vi "Main.vi"() -> ()   [LabVIEW 2018]
panel:
  out "Array":dbl[](array[numeric])
  out "Cont em Seg":dbl caption="Contador em Segundos"
  out "Regressive Timer":i32
  out "Case Indicator":i8
  out "Cont Min":dbl caption="Contador em Minutos"
  in  "stop":bool
  out "Barramento":string
  in  "Tab Control":T1(tab)
  in  "Rampa 1":i8=50 min=0 max=80 step=1
  in  "Fechamento \nde Enzimas":i8 min=0 max=80 step=1
  in  "Iniciar":bool
  in  "Min L3":i32 min=0 step=1
  in  "Min L2":i32 min=0 step=1
  in  "Min L1":i32 min=0 step=1
  in  "Min Ferv":i32 min=0 step=1
  in  "Qt de \nLupulos":i8 min=0 max=3 step=1
  in  "Min FE":i32 min=0 step=1
  in  "Min R4":i32 min=0 step=1
  in  "Min R3":i32 min=0 step=1
  in  "Min R2":i32 min=0 step=1
  in  "Min R1":i32 min=0 step=1
  in  "Qt de Rampas":i8 min=0 max=4 step=1
  in  "Rampa 4":i8 min=0 max=80 step=1
  in  "Rampa 3":i8 min=0 max=80 step=1
  in  "Rampa 2":i8 min=0 max=80 step=1
  out "Waveform Graph":dbl[](graph)
  in  "Set B1":bool
  in  "Chv Manual Most":bool
  in  "Slide Pot Most":i8(slide)=19 min=0 max=100 scale=0.0..100.0
  out "Led Manual Most":bool
  out "Seg Prox R":i8
  out "Min Prox R":i8
  out "Status Misturador Most":bool
  out "Porcent Pot Most":dbl
  out "Rampa Atual":string
  out "SetPoint Temp":dbl
  out "Seg Most":dbl
  out "Min Most":dbl
  out "Hora Most":dbl
  out "Watts Pot Most":dbl
  out "Thermometer Most":dbl(slide) caption="TMost" scale=0.0..100.0
  out "Status Resistencia Most":bool
  out "Lúpulo 1":bool
  out "Lúpulo 2":bool
  out "Lúpulo 3":bool
  out "Rampa 1":bool
  out "Rampa 2":bool
  out "Rampa 3":bool
  out "Rampa 4":bool
  out "Fech de Enzimas":bool
  out "Fervura":bool
  out "Transferência":bool
  out "Mosturação":bool
  out "Setup":bool
  in  "Iniciar 2":bool
  in  "Resistencia":bool
  in  "Misturador":bool
  in  "Bomba":bool
  in  "Set B2":bool
  out "Porcent Pot Ferv":dbl
  in  "Chv Manual Ferv":bool
  out "Led Manual Ferv":bool
  in  "Slide Pot Ferv":i8(slide) min=0 max=100 step=1 scale=0.0..100.0
  out "Thermometer Ferv":dbl(slide) scale=0.0..100.0
  out "Botão Lupulo 3":bool
  out "Botão Lupulo 2":bool
  out "Botão Lupulo 1":bool
  out "Status Resistencia Ferv":bool
  out "Watts Pot Ferv":dbl
  out "Min Prox L":i32
  out "Seg Prox L":i32
  out "Hora Ferv":dbl
  out "Min Ferv":dbl
  out "Seg Ferv":dbl
  # "Processo de cerveja artesanal automatizado"
  # "Rampas de Temperatura"
  # "Tempo nas respectivas rampas"
  # "Tempo de fervura"
  # "ºC"
  # "1ª Rampa :"
  # "Minutos"
  # "Minutos"
  # "ºC"
  # "Minutos"
  # "2ª Rampa :"
  # "Tempo dos lúpulos"
  # "Minutos"
  # "ºC"
  # "Minutos"
  # "3ª Rampa :"
  # "Minutos"
  # "ºC"
  # "Minutos"
  # "4ª Rampa :"
  # "Rampas Temperatura"
  # "Minutos"
  # "Fechamento Enzimas :"
  # "Quantidade de Lúpulos"
  # "ºC"
  # "Minutos"
  # "Controle Manual"
  # "Temperatura (ºC)"
  # "Controle Supervisório :"
  # "Misturador :"
  # "Resistência :"
  # "Potência da Resistência :"
  # "W"
  # "Porcentagem Potência :"
  # "%"
  # "Rampa atual :"
  # "Valor da Rampa Atual :"
  # "ºC"
  # "Tempo p/ próxima rampa :"
  # "m"
  # "s"
  # "Tempo de Processo :"
  # "h"
  # "m"
  # "s"
  # "Bomba de Recirculação"
  # "Misturador"
  # "Resistência"
  # "Etapas Fervura"
  # "Etapas Mosturação"
  # "Processo Atual"
  # "Controle Manual"
  # "Controle Supervisório :"
  # "Temperatura (ºC)"
  # "Resistência :"
  # "Potência da Resistência :"
  # "W"
  # "Porcentagem Potência :"
  # "%"
  # "Lúpulo 1"
  # "Lúpulo 2"
  # "Lúpulo 3"
  # "Tempo p/ próximo lúpulo :"
  # "m"
  # "s"
  # "Tempo de Processo :"
  # "s"
  # "m"
  # "h"
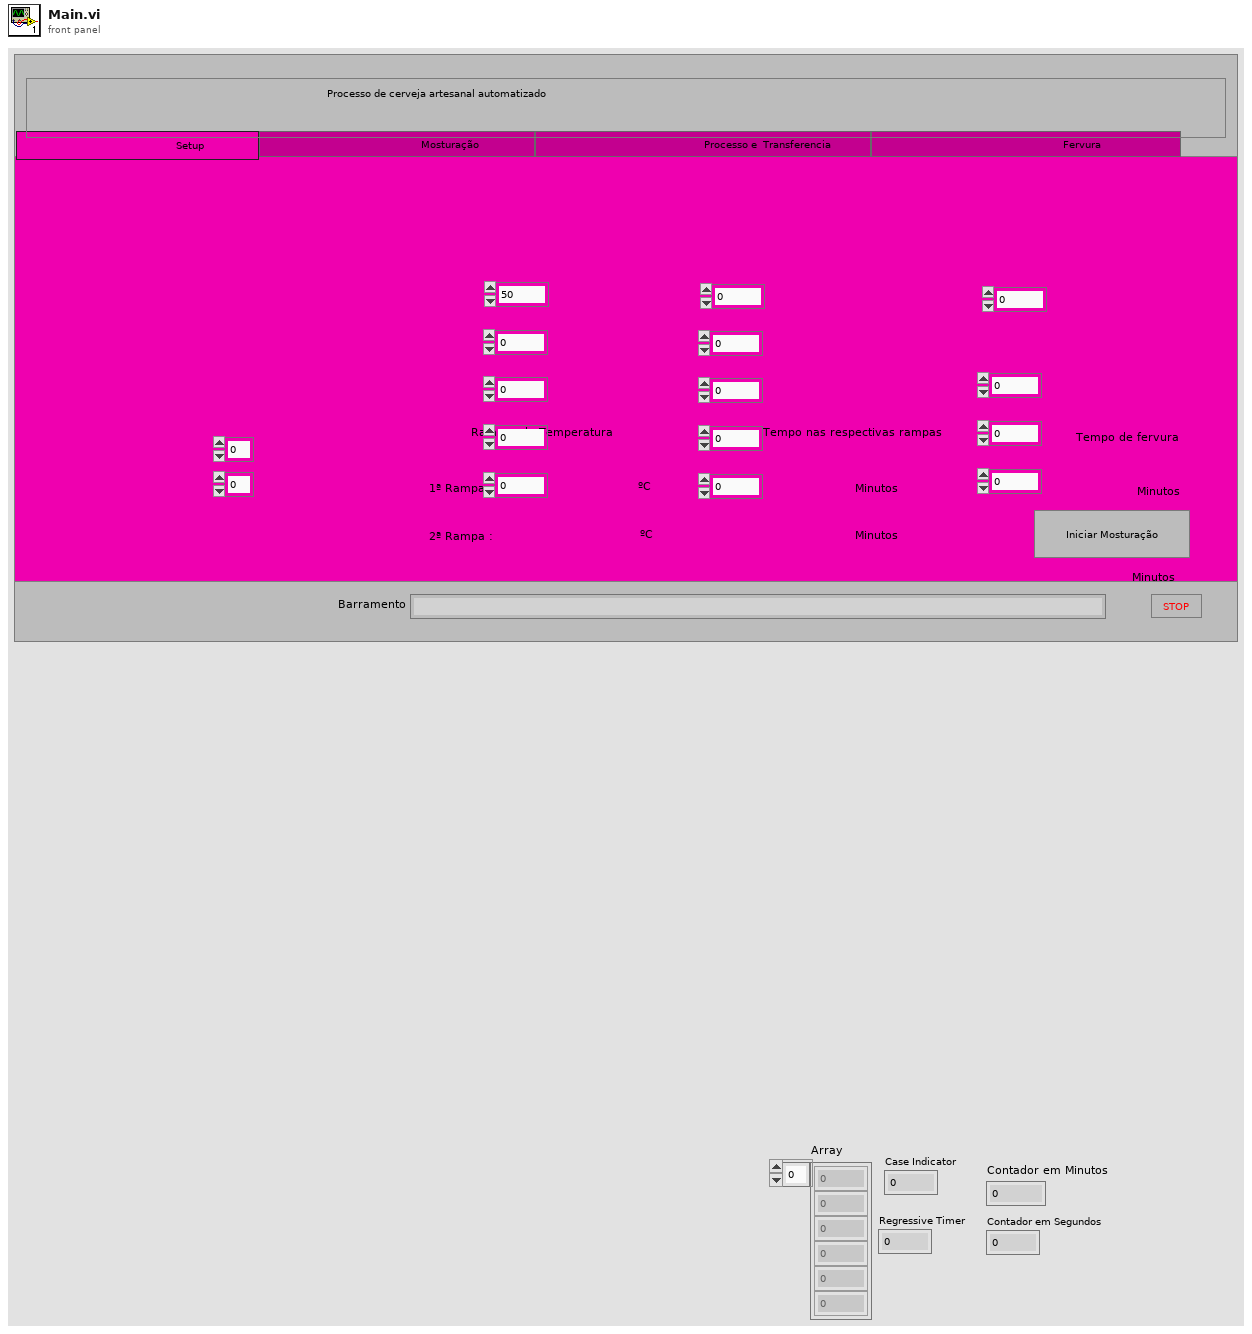
[diagram p1: front panel]
types:
  T1 = enum32{"                                   Setup                                ", "                                   Mosturação                                 ", "                                           Processo e  Transferencia                      ", "                                     Fervura                                                 "}
  T2 = typedef "LVDateTimeRec.ctl" = cluster{"fractional second":dbl, "second":i32, "minute":i32, "hour":i32, "day of month":i32, "month":i32, "year":i32, "day of week":i32, "day of year":i32, "DST":i32}
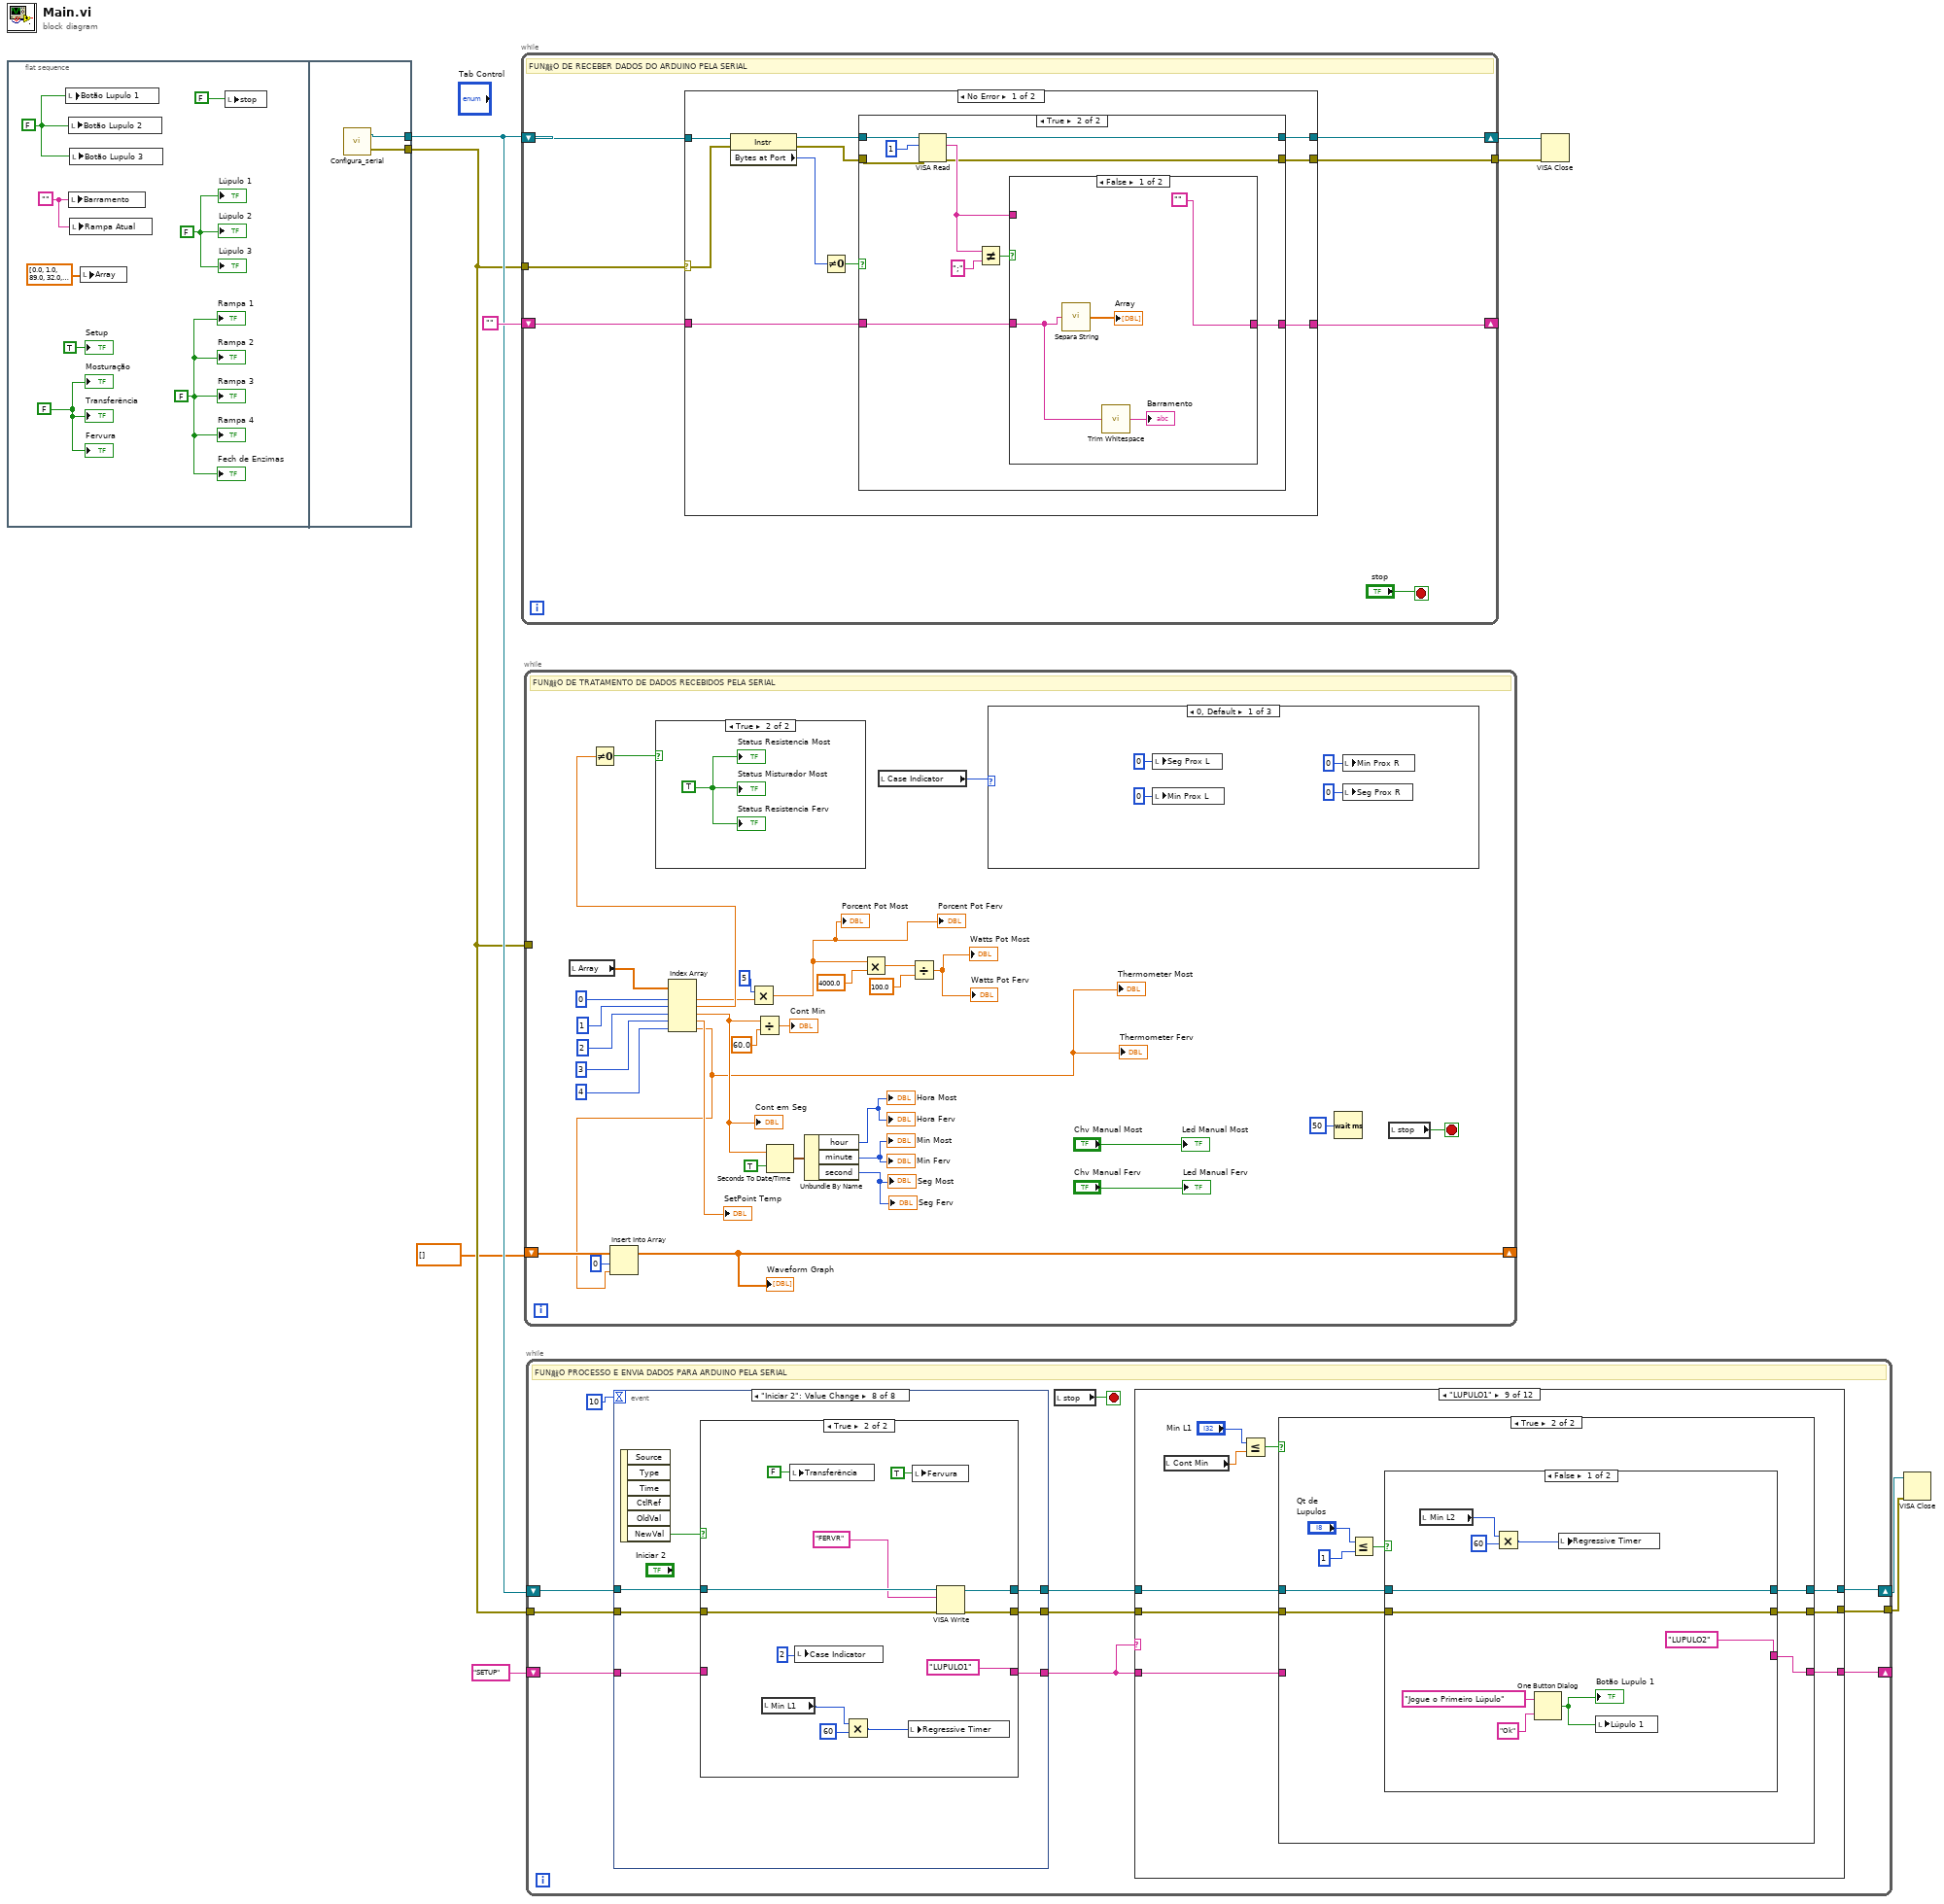
[diagram p0: block diagram]
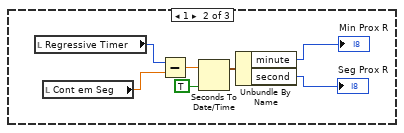
[diagram p2: hidden frame]
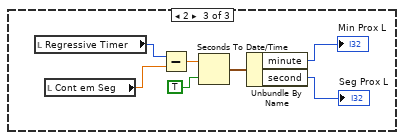
[diagram p3: hidden frame]
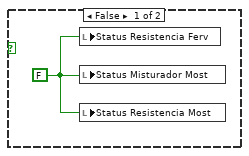
[diagram p4: hidden frame]
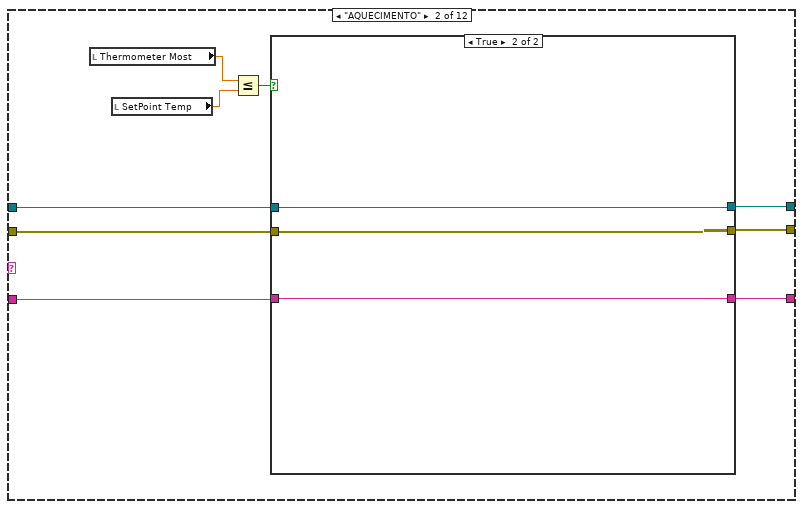
[diagram p6: hidden frame]
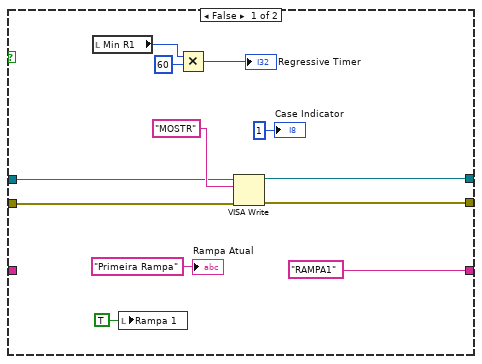
[diagram p7: hidden frame]
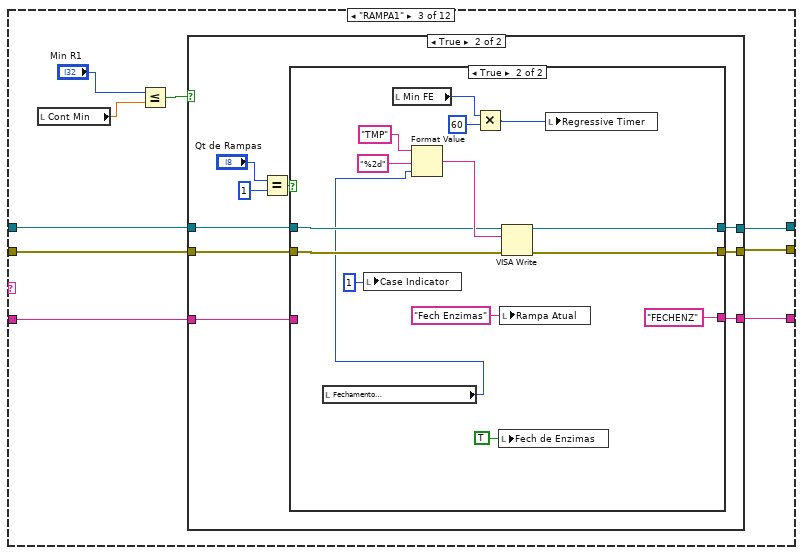
[diagram p8: hidden frame]
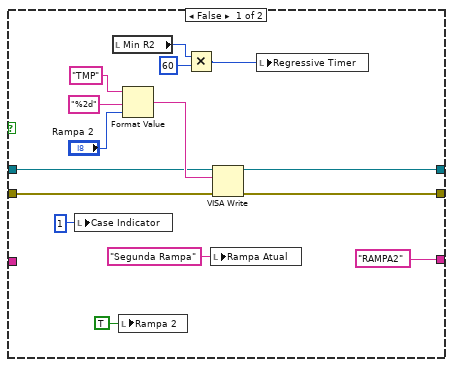
[diagram p10: hidden frame]
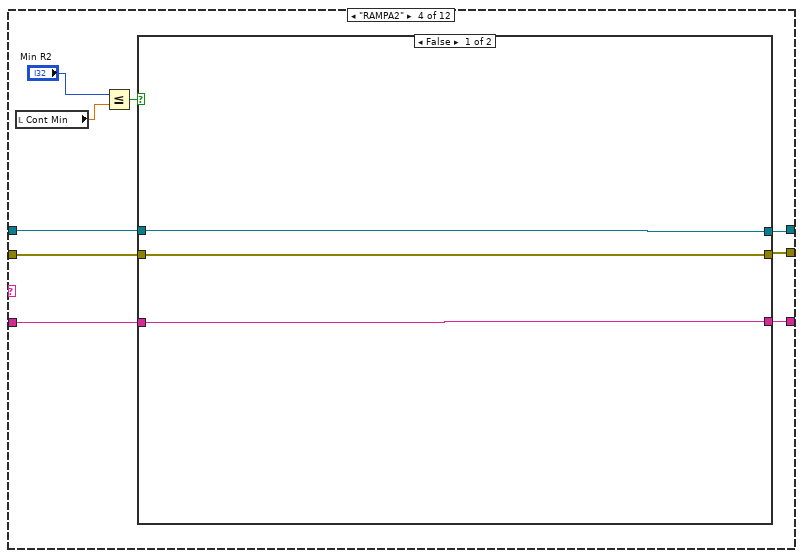
[diagram p11: hidden frame]
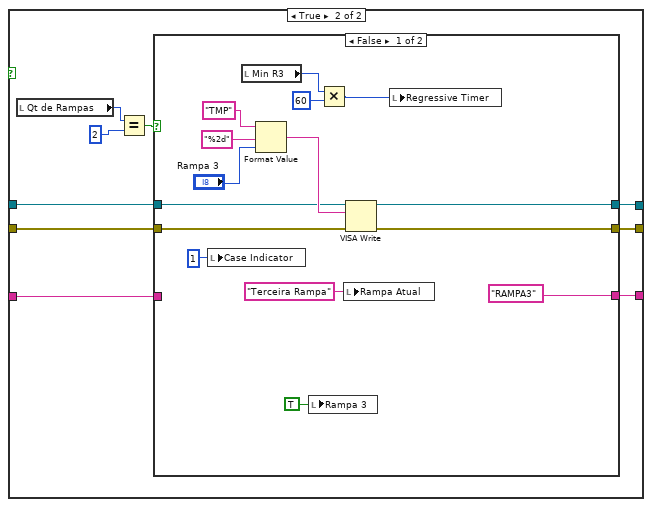
[diagram p12: hidden frame]
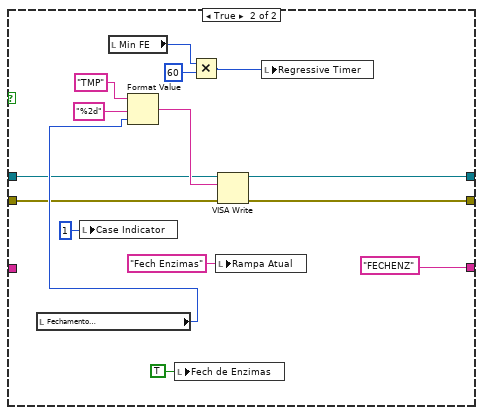
[diagram p13: hidden frame]
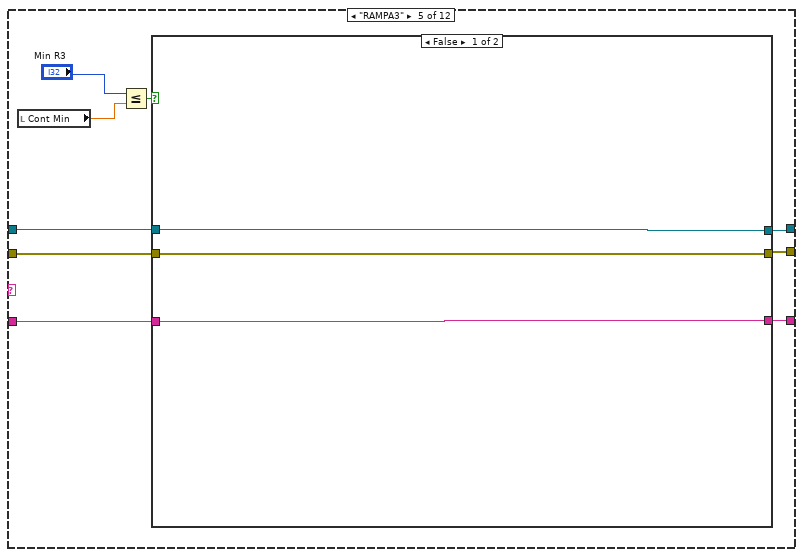
[diagram p14: hidden frame]
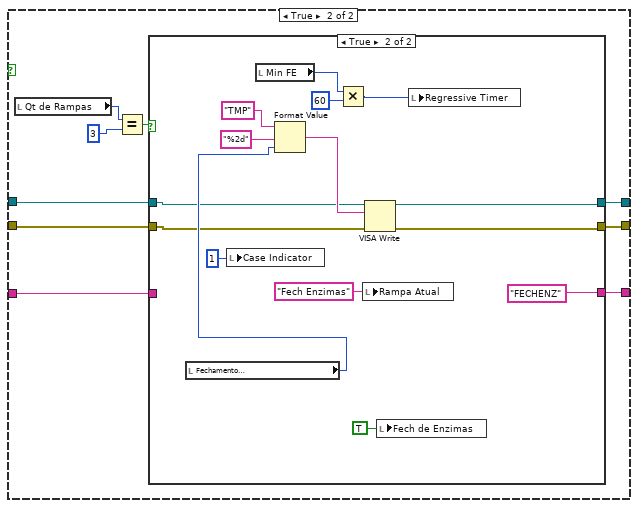
[diagram p15: hidden frame]
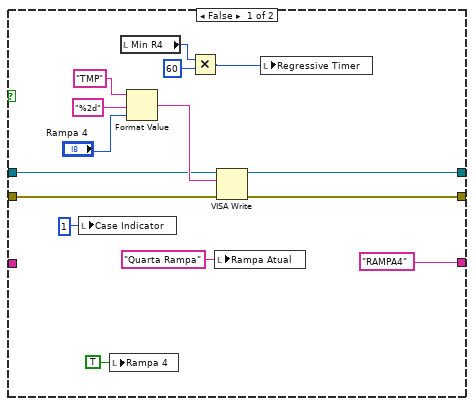
[diagram p16: hidden frame]
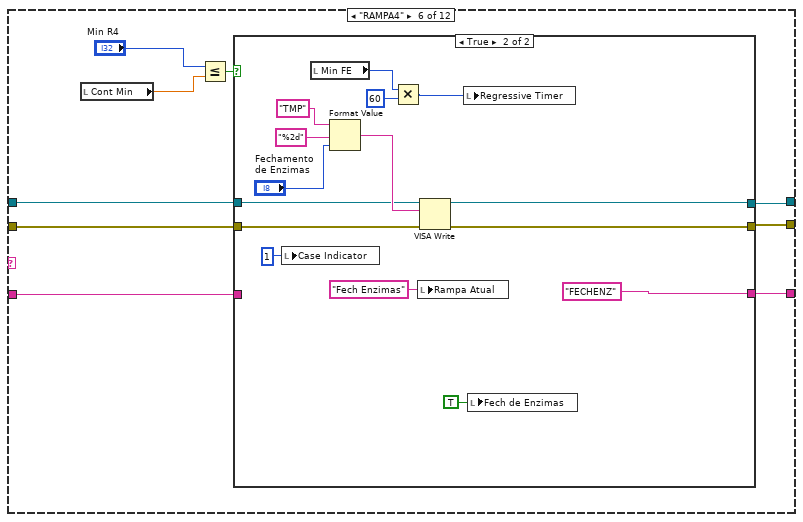
[diagram p17: hidden frame]
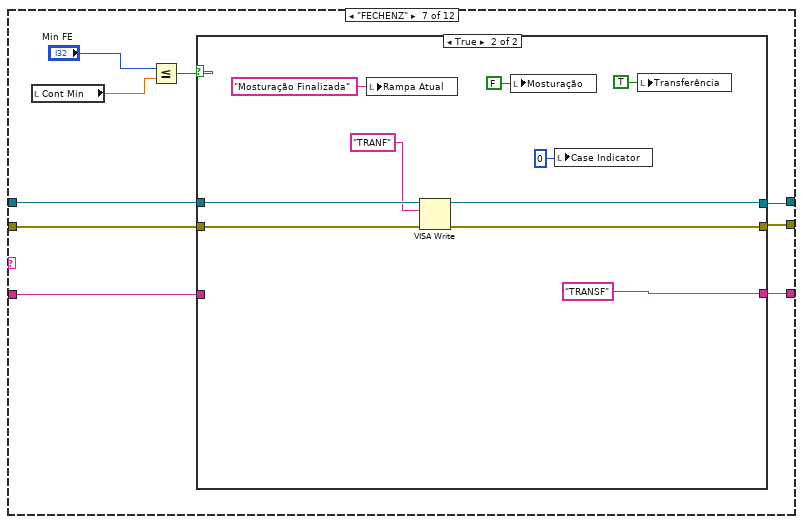
[diagram p19: hidden frame]
diagram:
  n1 = flat-sequence {
    tunnel: [w19] -> w5
    tunnel: [w18] -> w4
    frame #0 {
      w10 = FALSE
      w11 = FALSE ("Rampa 3")
      w12 = FALSE ("Rampa 3")
      w13 = FALSE
      w16 = ""
      n2 = local write "Botão Lupulo 1"(w10) -> ()
      n3 = local write "Botão Lupulo 2"(w10) -> ()
      n4 = local write "Barramento"(w16) -> ()
      n5 = local write "Botão Lupulo 3"(w10) -> ()
      n6 = local write "Rampa Atual"(w16) -> ()
      n7 = local write "Array"(dbl[] [0.0, 1.0, 89.0, 32.0, 24.93, 3.0, 0.0, 0.0, 0.0, 0.0, 0.0, 0.0, 0.0, 0.0, 0.0, 0.0, 0.0, 0.0, 0.0, 0.0] ("Array")) -> ()
      n8 = local write "stop"(FALSE) -> ()
      "Mosturação" <- w13
      "Setup" <- TRUE ("Setup")
      "Transferência" <- w13
      "Fervura" <- w13
      "Rampa 4" <- w12
      "Rampa 3" <- w12
      "Fech de Enzimas" <- w12
      "Rampa 2" <- w12
      "Rampa 1" <- w12
      "Lúpulo 3" <- w11
      "Lúpulo 2" <- w11
      "Lúpulo 1" <- w11
    }
    frame #1 {
      n9 = call "Configura_serial.vi"() -> ("VISA resource name out"=w19:refnum<visa-resource-name>, "error out"=w18:errorcluster)  [unwired: 1 in]
    }
  }
  n10 = while {
    shift-right: [w24] -> w8
    shift-left: w5 -> [w22]
    tunnel: w4 -> [w21]
    shift-right: [w25] -> _
    shift-left: "" -> [w26]
    tunnel: [w23] -> w7
    stop <- "stop" stop-if-true
    # "FUN敲O DE RECEBER DADOS DO ARDUINO PELA SERIAL"
    n11 = case shown="No Error" w21 {
      selector: w21 -> [w35 w57]
      tunnel: w22 -> [w36 w58]
      tunnel: w26 -> [w30 w59]
      tunnel: [w29 w59] -> w25
      tunnel: [w28 w58] -> w24
      tunnel: [w27 w57] -> w23
      frame No Error {
        n12 = property class="Instr"(reference=w36, error in=w35) -> (reference out=w32:refnum<visa-resource-name>, error out=w31:errorcluster, "Bytes at Port"=w34:u32)
        n13 = Not Equal To 0?(x=w34) -> (x != 0?=w33:bool)
        n14 = case shown="True" w33 {
          tunnel: w32 -> [w39 w49]
          tunnel: w31 -> [w38 w48]
          tunnel: w30 -> [w37 w43]
          tunnel: [w37 w42] -> w29
          tunnel: [w39 w41] -> w28
          tunnel: [w38 w40] -> w27
          frame False {
          }
          frame True {
            n15 = VISA Read(VISA resource name=w49, byte count=u32 1, error in (no error)=w48) -> (VISA resource name out=w41:refnum<visa-resource-name>, read buffer=w44:string, error out=w40:errorcluster)  [unwired: 1 out]
            n16 = Not Equal?(x=w44, y=";") -> (x != y?=w45:bool)
            n17 = case shown="False" w45 {
              tunnel: w44 -> [_ w55]
              tunnel: w43 -> [w51 w56]
              tunnel: ["" w54] -> w42
              frame False {
                n18 = call "Separa String.vi"("TEXTO DE ENTRADA"=w51) -> ("VETOR"=→"Array":dbl[])
                n19 = call <vilib>:"Trim Whitespace.vi"("string"=w51) -> ("trimmed string"=→"Barramento":string)  [unwired: 1 in]
              }
              frame True {
                n20 = Concatenate Strings(w56, w55) -> (w54:string)
              }
            }
          }
        }
      }
      frame Error {
      }
    }
  }
  n21 = while {
    tunnel: w4 -> [_]
    shift-right: [w60] -> _
    shift-left: dbl[] [] -> [w63]
    stop <- w83 stop-if-true
    # "FUN敲O DE TRATAMENTO DE DADOS RECEBIDOS PELA SERIAL"
    n22 = local read "Array"() -> (w69:dbl[])
    n23 = Index Array(array=w69, index #1=0, index #2=1, index #3=2, index #4=3 ("index"), index #5=4 ("index")) -> (element #1=w67:dbl, element #2=w86:dbl, element #3=w68:dbl, element #4=→"SetPoint Temp":dbl, element #5=w61:dbl)
    "Thermometer Most" <- w61
    "Thermometer Ferv" <- w61
    "Cont em Seg" <- w68
    n24 = Not Equal To 0?(x=w86) -> (x != 0?=w85:bool)
    n25 = Insert Into Array(array=w63, index=0, new element=w61) -> (w60:dbl[])
    "Waveform Graph" <- w60
    n26 = case shown="True" w85 {
      frame False {
        w111 = FALSE
        n27 = local write "Status Resistencia Ferv"(w111) -> ()
        n28 = local write "Status Misturador Most"(w111) -> ()
        n29 = local write "Status Resistencia Most"(w111) -> ()
      }
      frame True {
        w112 = TRUE
        "Status Resistencia Most" <- w112
        "Status Misturador Most" <- w112
        "Status Resistencia Ferv" <- w112
      }
    }
    n30 = Multiply(x=5, y=w67) -> (x*y=w82:dbl)
    "Porcent Pot Most" <- w82
    "Porcent Pot Ferv" <- w82
    n31 = Divide(x=w68, y=60.0) -> (x/y=→"Cont Min":dbl)
    n32 = Seconds To Date/Time(time stamp (now)=w68, to UTC (F)=TRUE) -> (date time rec=w72:T2)
    n33 = Unbundle By Name(w72) -> ("hour"=→"Hora Most" →"Hora Ferv":i32, "minute"=→"Min Most" →"Min Ferv":i32, "second"=→"Seg Most" →"Seg Ferv":i32)
    n34 = Multiply(x=w82, y=4000.0) -> (x*y=w80:dbl)
    n35 = local read "Case Indicator"() -> (w84:i8)
    n36 = Divide(x=w80, y=100.0) -> (x/y=→"Watts Pot Most" →"Watts Pot Ferv":dbl)
    n37 = case shown="0, Default" w84 {
      frame 0, Default {
        n38 = local write "Seg Prox L"(0 ("Seg Prox L")) -> ()
        n39 = local write "Min Prox L"(0 ("Min Prox L")) -> ()
        n40 = local write "Min Prox R"(i8 0 ("Min Prox R")) -> ()
        n41 = local write "Seg Prox R"(i8 0 ("Seg Prox R")) -> ()
      }
      frame 1 {
        n42 = local read "Regressive Timer"() -> (w103:i32)
        n43 = local read "Cont em Seg"() -> (w102:dbl)
        n44 = Subtract(x=w103, y=w102) -> (x-y=w98:dbl)
        n45 = Seconds To Date/Time(time stamp (now)=w98, to UTC (F)=TRUE) -> (date time rec=w101:T2)
        n46 = Unbundle By Name(w101) -> ("minute"=→"Min Prox R":i32, "second"=→"Seg Prox R":i32)
      }
      frame 2 {
        n47 = local read "Regressive Timer"() -> (w108:i32)
        n48 = local read "Cont em Seg"() -> (w107:dbl)
        n49 = Subtract(x=w108, y=w107) -> (x-y=w110:dbl)
        n50 = Seconds To Date/Time(time stamp (now)=w110, to UTC (F)=TRUE) -> (date time rec=w109:T2)
        n51 = Unbundle By Name(w109) -> ("minute"=→"Min Prox L":i32, "second"=→"Seg Prox L":i32)
      }
    }
    n52 = Wait (ms)(milliseconds to wait=u32 50) -> ()  [unwired: 1 out]
    n53 = local read "stop"() -> (w83:bool)
    "Led Manual Ferv" <- "Chv Manual Ferv"
    "Led Manual Most" <- "Chv Manual Most"
  }
  n54 = while {
    tunnel: w4 -> [w122]
    shift-right: [w118] -> _
    shift-left: "SETUP" -> [w120]
    shift-right: [w114] -> w3
    shift-left: w5 -> [w115]
    tunnel: [w113] -> w2
    stop <- w121 stop-if-true
    # "FUN敲O PROCESSO E ENVIA DADOS PARA ARDUINO PELA SERIAL"
    n55 = event shown="[7] \"Iniciar 2\": Value Change" {
      selector: _ -> [_ _ _ _ _ _ _ _]
      dyn-events: _ -> [_ _ _ _ _ _ _ _]
      timeout: 10 -> [_ _ _ _ _ _ _ _]
      tunnel: w115 -> [w467 w475 w496 w508 w520 w536 w552 w569]
      tunnel: w122 -> [w466 w474 w495 w507 w519 w535 w551 w568]
      tunnel: w120 -> [w468 w469 w493 w505 w515 w531 w547 w565]
      tunnel: [w468 w470 w493 w505 w515 w531 w547 w566] -> w119
      tunnel: [w467 w472 w492 w504 w517 w533 w549 w564] -> w117
      tunnel: [w466 w471 w491 w503 w516 w532 w548 w563] -> w116
      event Timeout {
        n56 = event-data() -> ()  [unwired: 1 in, 3 out]
      }
      event "Iniciar": Value Change {
        n57 = event-data() -> ("NewVal"=w473:bool)  [unwired: 1 in, 5 out]
        n58 = case shown="True" w473 {
          tunnel: w475 -> [w478 w490]
          tunnel: w474 -> [w477 w489]
          tunnel: [w478 w485] -> w472
          tunnel: [w477 w484] -> w471
          tunnel: [w476 "AQUECIMENTO"] -> w470
          tunnel: w469 -> [w476 _]
          frame False {
          }
          frame True {
            n59 = local write "Mosturação"(TRUE ("Mosturação")) -> ()
            n60 = local write "Setup"(FALSE ("Setup")) -> ()
            n61 = local write "Rampa Atual"("Aquecendo" ("Rampa Atual")) -> ()
            n62 = Format Value(string ("")="AQC", format string="%2d", value (0)="Rampa 1") -> (output string=w486:string)
            n63 = VISA Write(VISA resource name=w490, write buffer=w486, error in (no error)=w489) -> (VISA resource name out=w485:refnum<visa-resource-name>, error out=w484:errorcluster)  [unwired: 1 out]
          }
        }
      }
      event "Set B1": Value Change {
        n64 = event-data() -> ()  [unwired: 1 in, 6 out]
        n65 = Divide(x="Slide Pot Most", y=i8 5) -> (x/y=w498:dbl)
        n66 = To Byte Integer(number=w498) -> (8bit integer=w497:i8)
        n67 = Format Value(string ("")="POT", format string="%2d", value (0)=w497) -> (output string=w501:string)
        n68 = VISA Write(VISA resource name=w496, write buffer=w501, error in (no error)=w495) -> (VISA resource name out=w492:refnum<visa-resource-name>, error out=w491:errorcluster)  [unwired: 1 out]
      }
      event "Set B2": Value Change {
        n69 = event-data() -> ()  [unwired: 1 in, 6 out]
        n70 = Divide(x="Slide Pot Ferv", y=i8 5) -> (x/y=w510:dbl)
        n71 = To Byte Integer(number=w510) -> (8bit integer=w509:i8)
        n72 = Format Value(string ("")="POT", format string="%2d", value (0)=w509) -> (output string=w513:string)
        n73 = VISA Write(VISA resource name=w508, write buffer=w513, error in (no error)=w507) -> (VISA resource name out=w504:refnum<visa-resource-name>, error out=w503:errorcluster)  [unwired: 1 out]
      }
      event "Bomba": Value Change {
        n74 = event-data() -> ("NewVal"=w518:bool)  [unwired: 1 in, 5 out]
        n75 = case shown="False" w518 {
          tunnel: w520 -> [w525 w530]
          tunnel: w519 -> [w524 w529]
          tunnel: [w522 w527] -> w517
          tunnel: [w521 w526] -> w516
          frame False {
            n76 = VISA Write(VISA resource name=w525, write buffer="DSLGB", error in (no error)=w524) -> (VISA resource name out=w522:refnum<visa-resource-name>, error out=w521:errorcluster)  [unwired: 1 out]
          }
          frame True {
            n77 = VISA Write(VISA resource name=w530, write buffer="LIGAB", error in (no error)=w529) -> (VISA resource name out=w527:refnum<visa-resource-name>, error out=w526:errorcluster)  [unwired: 1 out]
          }
        }
      }
      event "Misturador": Value Change {
        n78 = event-data() -> ("NewVal"=w534:bool)  [unwired: 1 in, 5 out]
        n79 = case shown="False" w534 {
          tunnel: w536 -> [w541 w546]
          tunnel: w535 -> [w540 w545]
          tunnel: [w538 w543] -> w533
          tunnel: [w537 w542] -> w532
          frame False {
            n80 = VISA Write(VISA resource name=w541, write buffer="DSLGM", error in (no error)=w540) -> (VISA resource name out=w538:refnum<visa-resource-name>, error out=w537:errorcluster)  [unwired: 1 out]
          }
          frame True {
            n81 = VISA Write(VISA resource name=w546, write buffer="LIGAM", error in (no error)=w545) -> (VISA resource name out=w543:refnum<visa-resource-name>, error out=w542:errorcluster)  [unwired: 1 out]
          }
        }
      }
      event "Resistencia": Value Change {
        n82 = event-data() -> ("NewVal"=w550:bool)  [unwired: 1 in, 5 out]
        n83 = case shown="True" w550 {
          tunnel: w552 -> [w557 w562]
          tunnel: w551 -> [w556 w561]
          tunnel: [w554 w559] -> w549
          tunnel: [w553 w558] -> w548
          frame False {
            n84 = VISA Write(VISA resource name=w557, write buffer="DSLGR", error in (no error)=w556) -> (VISA resource name out=w554:refnum<visa-resource-name>, error out=w553:errorcluster)  [unwired: 1 out]
          }
          frame True {
            n85 = VISA Write(VISA resource name=w562, write buffer="LIGAR", error in (no error)=w561) -> (VISA resource name out=w559:refnum<visa-resource-name>, error out=w558:errorcluster)  [unwired: 1 out]
          }
        }
      }
      event "Iniciar 2": Value Change {
        n86 = event-data() -> ("NewVal"=w567:bool)  [unwired: 1 in, 5 out]
        n87 = case shown="True" w567 {
          tunnel: w569 -> [w571 w584]
          tunnel: w568 -> [w570 w583]
          tunnel: [w572 "LUPULO1"] -> w566
          tunnel: w565 -> [w572 _]
          tunnel: [w571 w578] -> w564
          tunnel: [w570 w577] -> w563
          frame False {
          }
          frame True {
            n88 = local read "Min L1"() -> (w579:i32)
            n89 = local write "Transferência"(FALSE ("Transferência")) -> ()
            n90 = local write "Case Indicator"(i8 2 ("Case Indicator")) -> ()
            n91 = Multiply(x=w579, y=60 ("x/y")) -> (x*y=w573:i32)
            n92 = local write "Regressive Timer"(w573) -> ()
            n93 = local write "Fervura"(TRUE ("Fervura")) -> ()
            n94 = VISA Write(VISA resource name=w584, write buffer="FERVR", error in (no error)=w583) -> (VISA resource name out=w578:refnum<visa-resource-name>, error out=w577:errorcluster)  [unwired: 1 out]
          }
        }
      }
    }
    n95 = local read "stop"() -> (w121:bool)
    n96 = case shown="\"LUPULO1\"" w119 {
      tunnel: w119 -> [w124 w135 w155 w209 w258 w309 w336 w355 w361 w397 w433 w452]
      tunnel: [w124 w134 w156 w210 w259 w310 w337 w355 w362 w398 w434 w453] -> w118
      tunnel: w117 -> [w126 w133 w152 w206 w255 w306 w333 w353 w360 w396 w432 w451]
      tunnel: w116 -> [w125 w132 w154 w208 w257 w308 w335 w354 w358 w394 w430 w449]
      tunnel: [w126 w131 w151 w205 w254 w305 w332 w353 w359 w395 w431 w450] -> w114
      tunnel: [w125 w130 w153 w207 w256 w307 w334 w354 w357 w393 w429 w448] -> w113
      frame "SETUP", Default {
      }
      frame "AQUECIMENTO" {
        n97 = local read "Thermometer Most"() -> (w128:dbl)
        n98 = local read "SetPoint Temp"() -> (w127:dbl)
        n99 = Less Or Equal?(x=w128, y=w127) -> (x <= y?=w129:bool)
        n100 = case shown="True" w129 {
          tunnel: w135 -> [_ w150]
          tunnel: ["RAMPA1" w150] -> w134
          tunnel: w133 -> [w144 w149]
          tunnel: w132 -> [w143 w148]
          tunnel: [w142 w149] -> w131
          tunnel: [w141 w148] -> w130
          frame False {
            n101 = local read "Min R1"() -> (w140:i32)
            n102 = local write "Rampa 1"(TRUE ("Rampa 1")) -> ()
            n103 = Multiply(x=w140, y=60 ("x/y")) -> (x*y=→"Regressive Timer":i32)
            n104 = VISA Write(VISA resource name=w144, write buffer="MOSTR", error in (no error)=w143) -> (VISA resource name out=w142:refnum<visa-resource-name>, error out=w141:errorcluster)  [unwired: 1 out]
            "Rampa Atual" <- "Primeira Rampa" ("Rampa Atual")
            "Case Indicator" <- i8 1 ("Case Indicator")
          }
          frame True {
          }
        }
      }
      frame "RAMPA1" {
        n105 = local read "Cont Min"() -> (w158:dbl)
        n106 = Less Or Equal?(x="Min R1", y=w158) -> (x <= y?=w157:bool)
        n107 = case shown="True" w157 {
          tunnel: [w162 w164] -> w156
          tunnel: w155 -> [w162 w163]
          tunnel: [w161 w169] -> w153
          tunnel: w154 -> [w161 w170]
          tunnel: [w160 w168] -> w151
          tunnel: w152 -> [w160 w171]
          frame False {
          }
          frame True {
            n108 = Equal?(x="Qt de Rampas", y=i8 1) -> (x = y?=w167:bool)
            n109 = case shown="True" w167 {
              tunnel: w171 -> [w183 w195]
              tunnel: w170 -> [w182 w194]
              tunnel: [w181 w193] -> w169
              tunnel: [w180 w192] -> w168
              tunnel: ["RAMPA2" "FECHENZ"] -> w164
              tunnel: w163 -> [_ _]
              frame False {
                n110 = local write "Case Indicator"(i8 1 ("Case Indicator")) -> ()
                n111 = local read "Min R2"() -> (w176:i32)
                n112 = local write "Rampa 2"(TRUE ("Rampa 2")) -> ()
                n113 = Format Value(string ("")="TMP", format string="%2d", value (0)="Rampa 2") -> (output string=w184:string)
                n114 = Multiply(x=w176, y=60 ("x/y")) -> (x*y=w173:i32)
                n115 = local write "Rampa Atual"("Segunda Rampa" ("Rampa Atual")) -> ()
                n116 = VISA Write(VISA resource name=w183, write buffer=w184, error in (no error)=w182) -> (VISA resource name out=w180:refnum<visa-resource-name>, error out=w181:errorcluster)  [unwired: 1 out]
                n117 = local write "Regressive Timer"(w173) -> ()
              }
              frame True {
                n118 = local read "Fechamento \nde Enzimas"() -> (w191:i8)
                n119 = local write "Case Indicator"(i8 1 ("Case Indicator")) -> ()
                n120 = local read "Min FE"() -> (w200:i32)
                n121 = Format Value(string ("")="TMP", format string="%2d", value (0)=w191) -> (output string=w201:string)
                n122 = Multiply(x=w200, y=60 ("x/y")) -> (x*y=w188:i32)
                n123 = local write "Fech de Enzimas"(TRUE ("Fech de Enzimas")) -> ()
                n124 = local write "Rampa Atual"("Fech Enzimas" ("Rampa Atual")) -> ()
                n125 = VISA Write(VISA resource name=w195, write buffer=w201, error in (no error)=w194) -> (VISA resource name out=w192:refnum<visa-resource-name>, error out=w193:errorcluster)  [unwired: 1 out]
                n126 = local write "Regressive Timer"(w188) -> ()
              }
            }
          }
        }
      }
      frame "RAMPA2" {
        n127 = local read "Cont Min"() -> (w203:dbl)
        n128 = Less Or Equal?(x="Min R2", y=w203) -> (x <= y?=w202:bool)
        n129 = case shown="False" w202 {
          tunnel: [w213 w218] -> w210
          tunnel: w209 -> [w213 w214]
          tunnel: [w212 w220] -> w207
          tunnel: w208 -> [w212 w221]
          tunnel: [w211 w219] -> w205
          tunnel: w206 -> [w211 w222]
          frame False {
          }
          frame True {
            n130 = local read "Qt de Rampas"() -> (w217:i8)
            n131 = Equal?(x=w217, y=i8 2) -> (x = y?=w215:bool)
            n132 = case shown="False" w215 {
              tunnel: w222 -> [w234 w241]
              tunnel: w221 -> [w233 w242]
              tunnel: [w232 w243] -> w220
              tunnel: [w231 w244] -> w219
              tunnel: ["RAMPA3" "FECHENZ"] -> w218
              tunnel: w214 -> [_ _]
              frame False {
                n133 = local write "Case Indicator"(i8 1 ("Case Indicator")) -> ()
                n134 = local read "Min R3"() -> (w226:i32)
                n135 = Format Value(string ("")="TMP", format string="%2d", value (0)="Rampa 3") -> (output string=w235:string)
                n136 = local write "Rampa 3"(TRUE ("Rampa 3")) -> ()
                n137 = Multiply(x=w226, y=60 ("x/y")) -> (x*y=w224:i32)
                n138 = local write "Rampa Atual"("Terceira Rampa" ("Rampa Atual")) -> ()
                n139 = VISA Write(VISA resource name=w234, write buffer=w235, error in (no error)=w233) -> (VISA resource name out=w231:refnum<visa-resource-name>, error out=w232:errorcluster)  [unwired: 1 out]
                n140 = local write "Regressive Timer"(w224) -> ()
              }
              frame True {
                n141 = local read "Fechamento \nde Enzimas"() -> (w246:i8)
                n142 = local write "Case Indicator"(i8 1 ("Case Indicator")) -> ()
                n143 = local read "Min FE"() -> (w251:i32)
                n144 = Format Value(string ("")="TMP", format string="%2d", value (0)=w246) -> (output string=w252:string)
                n145 = local write "Fech de Enzimas"(TRUE ("Fech de Enzimas")) -> ()
                n146 = Multiply(x=w251, y=60 ("x/y")) -> (x*y=w239:i32)
                n147 = local write "Rampa Atual"("Fech Enzimas" ("Rampa Atual")) -> ()
                n148 = VISA Write(VISA resource name=w241, write buffer=w252, error in (no error)=w242) -> (VISA resource name out=w244:refnum<visa-resource-name>, error out=w243:errorcluster)  [unwired: 1 out]
                n149 = local write "Regressive Timer"(w239) -> ()
              }
            }
          }
        }
      }
      frame "RAMPA3" {
        n150 = local read "Cont Min"() -> (w261:dbl)
        n151 = Less Or Equal?(x="Min R3", y=w261) -> (x <= y?=w260:bool)
        n152 = case shown="False" w260 {
          tunnel: [w264 w269] -> w259
          tunnel: w258 -> [w264 w268]
          tunnel: [w263 w271] -> w256
          tunnel: w257 -> [w263 w272]
          tunnel: [w262 w270] -> w254
          tunnel: w255 -> [w262 w273]
          frame False {
          }
          frame True {
            n153 = local read "Qt de Rampas"() -> (w267:i8)
            n154 = Equal?(x=w267, y=i8 3) -> (x = y?=w265:bool)
            n155 = case shown="True" w265 {
              tunnel: w273 -> [w285 w296]
              tunnel: w272 -> [w284 w295]
              tunnel: [w283 w293] -> w271
              tunnel: [w282 w294] -> w270
              tunnel: ["RAMPA4" "FECHENZ"] -> w269
              tunnel: w268 -> [_ _]
              frame False {
                n156 = local write "Case Indicator"(i8 1 ("Case Indicator")) -> ()
                n157 = local write "Rampa 4"(TRUE ("Rampa 4")) -> ()
                n158 = local read "Min R4"() -> (w276:i32)
                n159 = Format Value(string ("")="TMP", format string="%2d", value (0)="Rampa 4") -> (output string=w286:string)
                n160 = Multiply(x=w276, y=60 ("x/y")) -> (x*y=w275:i32)
                n161 = local write "Rampa Atual"("Quarta Rampa" ("Rampa Atual")) -> ()
                n162 = VISA Write(VISA resource name=w285, write buffer=w286, error in (no error)=w284) -> (VISA resource name out=w282:refnum<visa-resource-name>, error out=w283:errorcluster)  [unwired: 1 out]
                n163 = local write "Regressive Timer"(w275) -> ()
              }
              frame True {
                n164 = local read "Fechamento \nde Enzimas"() -> (w301:i8)
                n165 = local write "Case Indicator"(i8 1 ("Case Indicator")) -> ()
                n166 = local read "Min FE"() -> (w302:i32)
                n167 = Format Value(string ("")="TMP", format string="%2d", value (0)=w301) -> (output string=w303:string)
                n168 = Multiply(x=w302, y=60 ("x/y")) -> (x*y=w290:i32)
                n169 = local write "Rampa Atual"("Fech Enzimas" ("Rampa Atual")) -> ()
                n170 = VISA Write(VISA resource name=w296, write buffer=w303, error in (no error)=w295) -> (VISA resource name out=w294:refnum<visa-resource-name>, error out=w293:errorcluster)  [unwired: 1 out]
                n171 = local write "Fech de Enzimas"(TRUE ("Fech de Enzimas")) -> ()
                n172 = local write "Regressive Timer"(w290) -> ()
              }
            }
          }
        }
      }
      frame "RAMPA4" {
        n173 = local read "Cont Min"() -> (w312:dbl)
        n174 = Less Or Equal?(x="Min R4", y=w312) -> (x <= y?=w311:bool)
        n175 = case shown="True" w311 {
          tunnel: [w315 "FECHENZ"] -> w310
          tunnel: w309 -> [w315 _]
          tunnel: [w314 w325] -> w307
          tunnel: w308 -> [w314 w326]
          tunnel: [w313 w324] -> w305
          tunnel: w306 -> [w313 w327]
          frame False {
          }
          frame True {
            n176 = local write "Case Indicator"(i8 1 ("Case Indicator")) -> ()
            n177 = local read "Min FE"() -> (w319:i32)
            n178 = Format Value(string ("")="TMP", format string="%2d", value (0)="Fechamento \nde Enzimas") -> (output string=w328:string)
            n179 = Multiply(x=w319, y=60 ("x/y")) -> (x*y=w317:i32)
            n180 = local write "Rampa Atual"("Fech Enzimas" ("Rampa Atual")) -> ()
            n181 = VISA Write(VISA resource name=w327, write buffer=w328, error in (no error)=w326) -> (VISA resource name out=w324:refnum<visa-resource-name>, error out=w325:errorcluster)  [unwired: 1 out]
            n182 = local write "Regressive Timer"(w317) -> ()
            n183 = local write "Fech de Enzimas"(TRUE ("Fech de Enzimas")) -> ()
          }
        }
      }
      frame "FECHENZ" {
        n184 = local read "Cont Min"() -> (w339:dbl)
        n185 = Less Or Equal?(x="Min FE", y=w339) -> (x <= y?=w338:bool)
        n186 = case shown="True" w338 {
          tunnel: [w342 "TRANSF"] -> w337
          tunnel: w336 -> [w342 _]
          tunnel: [w341 w350] -> w334
          tunnel: w335 -> [w341 w351]
          tunnel: [w340 w349] -> w332
          tunnel: w333 -> [w340 w352]
          frame False {
          }
          frame True {
            n187 = local write "Rampa Atual"("Mosturação Finalizada" ("Rampa Atual")) -> ()
            n188 = VISA Write(VISA resource name=w352, write buffer="TRANF" ("Rampa Atual"), error in (no error)=w351) -> (VISA resource name out=w349:refnum<visa-resource-name>, error out=w350:errorcluster)  [unwired: 1 out]
            n189 = local write "Mosturação"(FALSE ("Mosturação")) -> ()
            n190 = local write "Case Indicator"(i8 0 ("Case Indicator")) -> ()
            n191 = local write "Transferência"(TRUE ("Transferência")) -> ()
          }
        }
      }
      frame "TRANSF" {
      }
      frame "LUPULO1" {
        n192 = local read "Cont Min"() -> (w364:dbl)
        n193 = Less Or Equal?(x="Min L1", y=w364) -> (x <= y?=w363:bool)
        n194 = case shown="True" w363 {
          tunnel: [w367 w375] -> w362
          tunnel: w361 -> [w367 _]
          tunnel: w360 -> [w366 w374]
          tunnel: [w366 w369] -> w359
          tunnel: w358 -> [w365 w373]
          tunnel: [w365 w368] -> w357
          frame False {
          }
          frame True {
            n195 = Less Or Equal?(x="Qt de \nLupulos", y=i8 1) -> (x <= y?=w372:bool)
            n196 = case shown="False" w372 {
              tunnel: ["LUPULO2" "FERVURA"] -> w375
              tunnel: w374 -> [w383 w390]
              tunnel: w373 -> [w382 w389]
              tunnel: [w383 w390] -> w369
              tunnel: [w382 w389] -> w368
              frame False {
                n197 = local read "Min L2"() -> (w376:i32)
                n198 = Multiply(x=w376, y=60 ("x/y")) -> (x*y=w378:i32)
                n199 = One Button Dialog(message="Jogue o Primeiro Lúpulo", button name ("OK")="Ok") -> (true=w379:bool)
                "Botão Lupulo 1" <- w379
                n200 = local write "Regressive Timer"(w378) -> ()
                n201 = local write "Lúpulo 1"(w379) -> ()
              }
              frame True {
                n202 = local write "Case Indicator"(i8 0 ("Case Indicator")) -> ()
                n203 = One Button Dialog(message="Jogue o Primeiro Lúpulo", button name ("OK")="Ok") -> (true=w386:bool)
                n204 = local write "Botão Lupulo 1"(w386) -> ()
                n205 = local write "Lúpulo 1"(w386) -> ()
              }
            }
          }
        }
      }
      frame "LUPULO2" {
        n206 = local read "Cont Min"() -> (w400:dbl)
        n207 = Less Or Equal?(x="Min L2", y=w400) -> (x <= y?=w399:bool)
        n208 = case shown="True" w399 {
          tunnel: [w403 w411] -> w398
          tunnel: w397 -> [w403 _]
          tunnel: w396 -> [w402 w410]
          tunnel: [w402 w406] -> w395
          tunnel: w394 -> [w401 w409]
          tunnel: [w401 w405] -> w393
          frame False {
          }
          frame True {
            n209 = local read "Qt de \nLupulos"() -> (w404:i8)
            n210 = Less Or Equal?(x=w404, y=i8 2) -> (x <= y?=w408:bool)
            n211 = case shown="True" w408 {
              tunnel: ["LUPULO3" "FERVURA"] -> w411
              tunnel: w410 -> [w419 w426]
              tunnel: w409 -> [w418 w425]
              tunnel: [w419 w426] -> w406
              tunnel: [w418 w425] -> w405
              frame False {
                n212 = local read "Min L3"() -> (w414:i32)
                n213 = One Button Dialog(message="Jogue o Segundo Lúpulo", button name ("OK")="Ok") -> (true=w415:bool)
                "Botão Lupulo 2" <- w415
                n214 = Multiply(x=w414, y=60 ("x/y")) -> (x*y=w413:i32)
                n215 = local write "Lúpulo 2"(w415) -> ()
                n216 = local write "Regressive Timer"(w413) -> ()
              }
              frame True {
                n217 = local write "Case Indicator"(i8 0 ("Case Indicator")) -> ()
                n218 = One Button Dialog(message="Jogue o Segundo Lúpulo", button name ("OK")="Ok") -> (true=w422:bool)
                n219 = local write "Botão Lupulo 2"(w422) -> ()
                n220 = local write "Lúpulo 2"(w422) -> ()
              }
            }
          }
        }
      }
      frame "LUPULO3" {
        n221 = local read "Cont Min"() -> (w436:dbl)
        n222 = Less Or Equal?(x="Min L3", y=w436) -> (x <= y?=w435:bool)
        n223 = case shown="True" w435 {
          tunnel: [w439 "FERVURA"] -> w434
          tunnel: w433 -> [w439 _]
          tunnel: w432 -> [w438 w445]
          tunnel: [w438 w445] -> w431
          tunnel: w430 -> [w437 w444]
          tunnel: [w437 w444] -> w429
          frame False {
          }
          frame True {
            n224 = local write "Case Indicator"(i8 0 ("Case Indicator")) -> ()
            n225 = One Button Dialog(message="Jogue o Terceiro Lúpulo", button name ("OK")="Ok") -> (true=w441:bool)
            "Botão Lupulo 3" <- w441
            n226 = local write "Lúpulo 3"(w441) -> ()
          }
        }
      }
      frame "FERVURA" {
        n227 = local read "Cont Min"() -> (w455:dbl)
        n228 = Less Or Equal?(x="Min Ferv", y=w455) -> (x <= y?=w454:bool)
        n229 = case shown="True" w454 {
          tunnel: [w458 "TRANSF"] -> w453
          tunnel: w452 -> [w458 _]
          tunnel: w451 -> [w457 w464]
          tunnel: [w457 w461] -> w450
          tunnel: w449 -> [w456 w463]
          tunnel: [w456 w460] -> w448
          frame False {
          }
          frame True {
            n230 = VISA Write(VISA resource name=w464, write buffer="FIMFV", error in (no error)=w463) -> (VISA resource name out=w461:refnum<visa-resource-name>, error out=w460:errorcluster)  [unwired: 1 out]
            n231 = local write "Fervura"(FALSE ("Fervura")) -> ()
          }
        }
      }
    }
  }
  n232 = VISA Close(VISA resource name=w8, error in (no error)=w7) -> ()  [unwired: 1 out]
  n233 = VISA Close(VISA resource name=w3, error in (no error)=w2) -> ()  [unwired: 1 out]
